vi "Set Point.vi"(8 "error in (no error)":errorcluster, 10 "Set point":dbl, 11 "Temperature Controller in":refnum<class "Temperature Controller.lvclass">) -> (0 "error out":errorcluster, 3 "Temperature Controller out":refnum<class "Temperature Controller.lvclass">)   [LabVIEW 2016, in "Temperature Controller.lvclass"]
uses:
  Temperature Controller.lvclass
  Read T ctl driver.vi
  Write T ctl driver.vi
  NHMFL_Core/Libraries/Instruments/Temperature Controller Driver/Temperature Controller Driver.lvclass
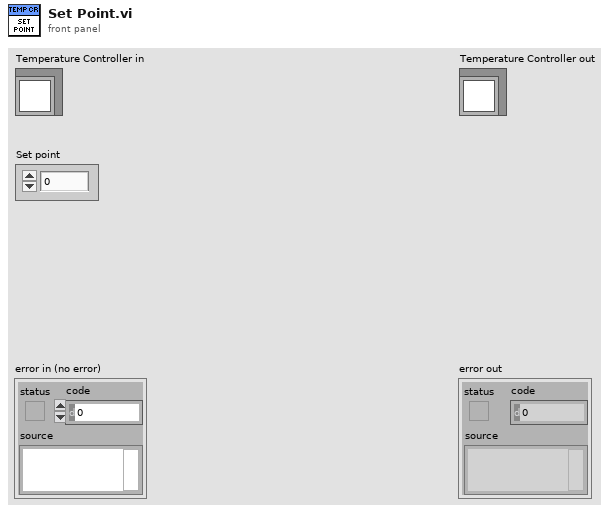
[diagram p1: front panel]
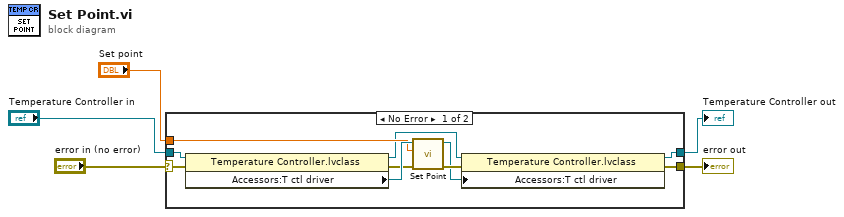
[diagram p0: block diagram]
diagram:
  n1 = case shown="No Error" "error in (no error)" {
    selector: "error in (no error)" -> [w15 w17]
    tunnel: [w11 w17] -> w4
    tunnel: [w9 w16] -> w2
    tunnel: "Temperature Controller in" -> [w14 w16]
    tunnel: "Set point" -> [w12 _]
    frame No Error {
      n2 = property class="Temperature Controller.lvclass"(reference=w14, error in=w15) -> (reference out=w10:refnum<class "Temperature Controller.lvclass">, error out=w8:errorcluster, "Accessors:T ctl driver"=w13:refnum<class "Temperature Controller Driver.lvclass">)
      n3 = call-dynamic "Set Point.vi"("error in (no error)"=w8, "Set point"=w12, "Temperature Controller Driver in"=w13) -> ("error out"=w7:errorcluster, "Temperature Controller Driver out"=w6:refnum<class "Temperature Controller Driver.lvclass">)  [unwired: 7 in]
      n4 = property class="Temperature Controller.lvclass"(reference=w10, error in=w7, "Accessors:T ctl driver"=w6) -> (reference out=w9:refnum<class "Temperature Controller.lvclass">, error out=w11:errorcluster)
    }
    frame Error {
    }
  }
  "error out" <- w4
  "Temperature Controller out" <- w2
